vi "Calibrate IMU Gyro.vi"(6 "Calib time (ms)":u32, 11 "I2CDevRef in":T1 {"Device Address" format="%.0x"}) -> (3 "I2CDevRef out":T1={"DevStatus"={"status"=FALSE, "code"=0, "source"=""}, "Device Address"=0, "Handle"=0, "I2C Bus"=enum."Invalid"} {"Device Address" format="%.0x"})   [LabVIEW 2015]
uses:
  <vilib>/Rock Robotics/WPI/I2C/WPI_I2CDevRef.ctl
  <vilib>/Rock Robotics/SystemInterfaces/i2clib/i2c_bus.ctl
  Robot Global Data.vi
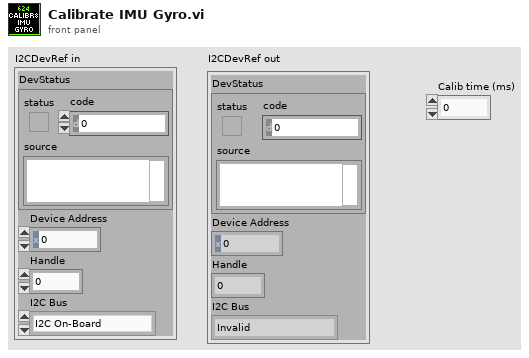
[diagram p1: front panel]
types:
  T1 = typedef "WPI_I2CDevRef.ctl" = cluster{"DevStatus":errorcluster, "Device Address":u8, "Handle":i32, "I2C Bus":T2}
  T2 = typedef "i2c_bus.ctl" = enum16{"I2C On-Board", "I2C MXP", "Invalid"}
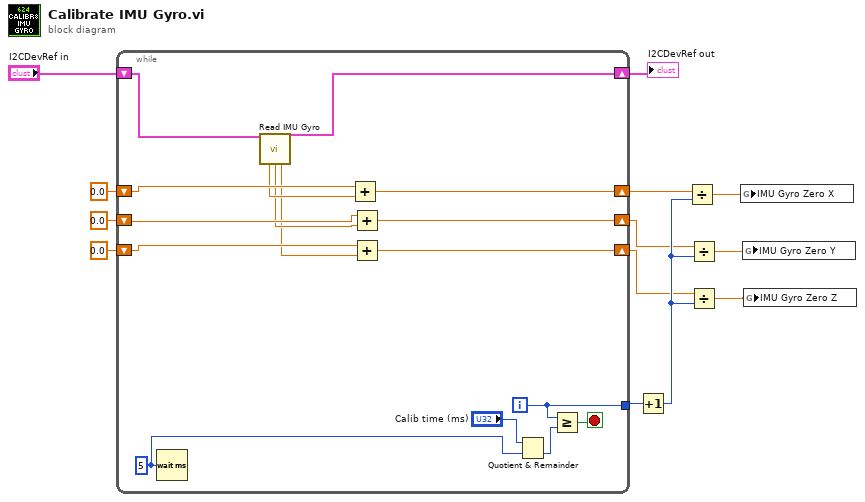
[diagram p0: block diagram]
diagram:
  n1 = while {
    shift-right: [w22] -> w12
    shift-left: "I2CDevRef in" -> [w23]
    tunnel: [w28] -> w10
    shift-right: [w21] -> w7
    shift-left: 0.0 -> [w24]
    shift-right: [w19] -> w6
    shift-left: 0.0 -> [w20]
    shift-right: [w18] -> w5
    shift-left: 0.0 -> [w17]
    i -> [w28]
    stop <- w29 stop-if-true
    w26 = u32 5 ("milliseconds to wait")
    n2 = Wait (ms)(milliseconds to wait=w26) -> ()  [unwired: 1 out]
    n3 = call "Read IMU Gyro.vi"("I2CDevRef"=w23) -> ("I2CDevRef 2"=w22:T1, "Raw X"=w16:dbl, "Raw Y"=w15:dbl, "Raw Z"=w14:dbl)  [unwired: 8 in, 3 out]
    n4 = Add(x=w24, y=w16) -> (x+y=w21:dbl)
    n5 = Add(x=w20, y=w15) -> (x+y=w19:dbl)
    n6 = Add(x=w17, y=w14) -> (x+y=w18:dbl)
    n7 = Quotient & Remainder(x="Calib time (ms)", y=w26) -> (floor(x/y)=w25:u32)  [unwired: 1 out]
    n8 = Greater Or Equal?(x=w28, y=w25) -> (x >= y?=w29:bool)
  }
  "I2CDevRef out" <- w12
  n9 = Increment(x=w10) -> (x+1=w8:i32)
  n10 = Divide(x=w7, y=w8) -> (x/y=w3:dbl)
  n11 = Divide(x=w6, y=w8) -> (x/y=w4:dbl)
  n12 = Divide(x=w5, y=w8) -> (x/y=w9:dbl)
  n13 = global write "Robot Global Data.vi" "IMU Gyro Zero X"(w3) -> ()
  n14 = global write "Robot Global Data.vi" "IMU Gyro Zero Y"(w4) -> ()
  n15 = global write "Robot Global Data.vi" "IMU Gyro Zero Z"(w9) -> ()
